vi "Motors Position Load.vi"(2 "error in":errorcluster, 3 "file path":path=path "C:/LabView VIs/IPES SubVIs/saved_positions.txt") -> (0 "error out":errorcluster, 1 "Positions":string[][](array[string]))   [LabVIEW 2018]
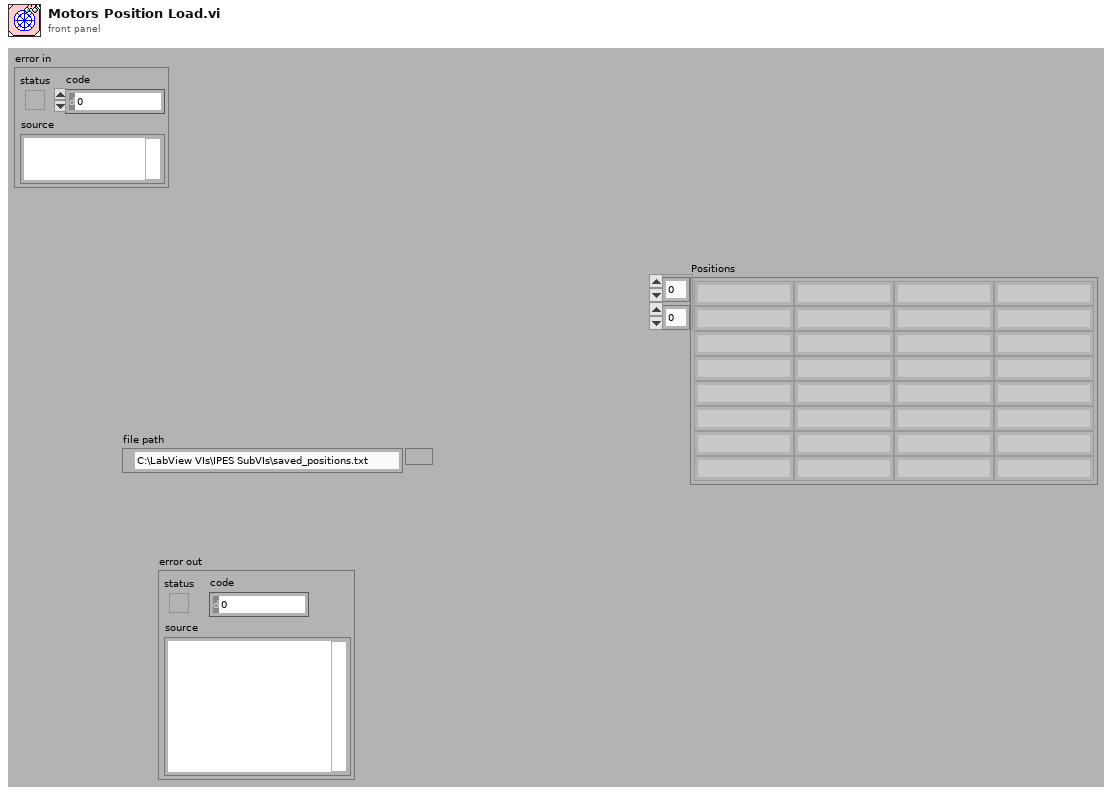
[diagram p1: front panel]
types:
  T1 = enum16{"open", "replace", "create", "open or create", "replace or create", "replace or create with confirmation"}
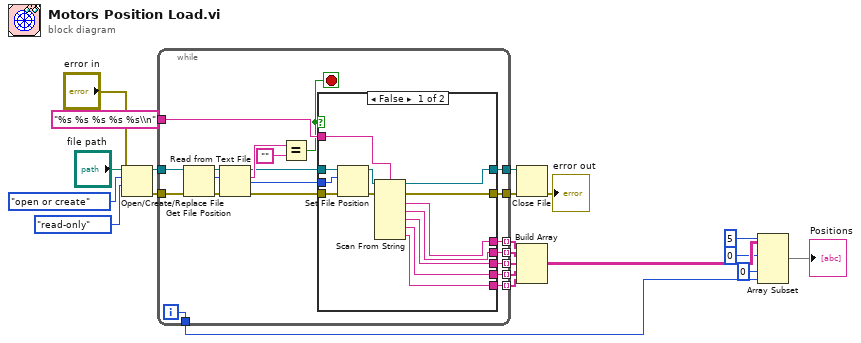
[diagram p0: block diagram]
diagram:
  n1 = Open/Create/Replace File(file path (use dialog)="file path", error in="error in", operation (0:open)=T1."open or create", access (0:read/write)=enum16{"read/write", "read-only", "write-only"}."read-only") -> (refnum out=w17:refnum<file>, error out=w13:errorcluster)  [unwired: 2 in, 1 out]
  n2 = while {
    tunnel: "%s %s %s %s %s\\n" ("format string") -> [w40]
    tunnel: w17 -> [w32]
    tunnel: [w33] -> w16
    tunnel: [w34] -> w14
    tunnel: w13 -> [w31]
    tunnel: [w35] -> w12 mode=indexing
    tunnel: [w39] -> w11 mode=indexing
    tunnel: [w38] -> w10 mode=indexing
    tunnel: [w37] -> w9 mode=indexing
    tunnel: [w36] -> w8 mode=indexing
    tunnel: [w22] -> w2
    i -> [w22]
    stop <- w26 stop-if-true
    n3 = Get File Position(4:w31, 7:w32) -> (0:w29:errorcluster, 2:w23:i64, 3:w30:refnum<file>)
    n4 = Read from Text File(file (use dialog)=w30, error in=w29) -> (refnum out=w25:refnum<file>, text=w27:string, error out=w24:errorcluster)  [unwired: 2 in, 1 out]
    n5 = Equal?(x=w27, y="") -> (x = y?=w26:bool)
    n6 = case shown="False" w26 {
      tunnel: w40 -> [w53 _]
      tunnel: [w52 _] -> w39
      tunnel: [w51 _] -> w38
      tunnel: [w50 _] -> w37
      tunnel: [w49 _] -> w36
      tunnel: [w48 _] -> w35
      tunnel: [w47 w55] -> w34
      tunnel: [w46 w54] -> w33
      tunnel: w25 -> [w45 w54]
      tunnel: w24 -> [w44 w55]
      tunnel: w23 -> [w41 _]
      frame False {
        n7 = Set File Position(offset (in bytes) (0)=w41, refnum=w45, error in=w44) -> (refnum out=w43:refnum<file>, error out=w42:errorcluster)  [unwired: 1 in]
        n8 = Scan From String(w53, w43, w42) -> (w46:refnum<file>, w47:errorcluster, output 1=w48:string, output 2=w52:string, output 3=w51:string, output 4=w50:string, output 5=w49:string)  [unwired: 5 in]
      }
      frame True {
      }
    }
  }
  n9 = Close File(refnum=w16, error in=w14) -> (error out=→"error out":errorcluster)  [unwired: 1 out]
  n10 = Build Array(w12, w11, w10, w9, w8) -> (w7:string[][])
  n11 = Array Subset(array=w7, index (row)=0 ("index"), length (row)=5 ("length"), index (col)=0 ("index"), length (col)=w2) -> (→"Positions":string[][])
